vi "Read Stream Data File Multiple Channel.vi"() -> ()   [LabVIEW 2020]
panel:
  out "Array":dbl[][](array[numeric])
  in  "Channel":u64
  out "Waveform Graph":dbl[][](graph)
  in  "File Path":path
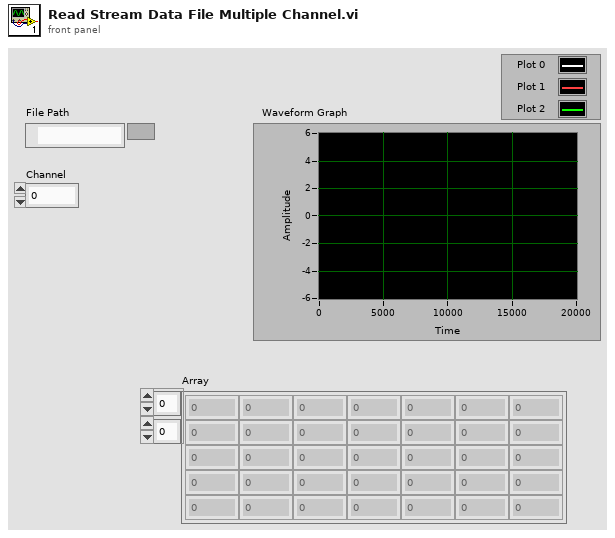
[diagram p1: front panel]
types:
  T1 = enum16{"open", "replace", "create", "open or create", "replace or create", "replace or create with confirmation"}
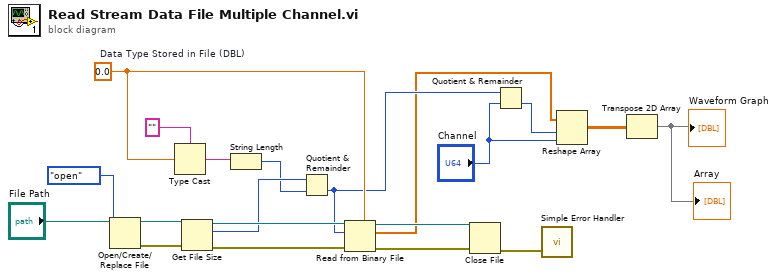
[diagram p0: block diagram]
diagram:
  w14 = 0.0  # Data Type Stored in File (DBL)
  n1 = Open/Create/Replace File(file path (use dialog)="File Path", operation (0:open)=T1."open") -> (refnum out=w18:refnum<file>, error out=w16:errorcluster)  [unwired: 4 in, 1 out]
  n2 = Type Cast(type="", x=w14) -> (*(type *) &x=w12:string)
  n3 = Get File Size(file=w18, error in=w16) -> (refnum out=w17:refnum<file>, size (in bytes)=w11:i64, 0:w15:errorcluster)
  n4 = String Length(string=w12) -> (length=w10:i32)
  n5 = Quotient & Remainder(x=w11, y=w10) -> (floor(x/y)=w6:i64)  [unwired: 1 out]
  n6 = Read from Binary File(5:w14, 8:w15, 10:w6, 11:w17) -> (0:w8:errorcluster, 2:w5:dbl[], 3:w9:refnum<file>)  [unwired: 2 in, 1 out]
  n7 = Close File(refnum=w9, error in=w8) -> (error out=w7:errorcluster)  [unwired: 1 out]
  n8 = Quotient & Remainder(x=w6, y="Channel") -> (floor(x/y)=w2:u64)  [unwired: 1 out]
  n9 = call <vilib>:"Simple Error Handler.vi"("error in (no error)"=w7) -> ()  [unwired: 4 in, 5 out]
  n10 = Reshape Array "Reshape Array"(w5, w2, "Channel") -> (w3:dbl[][])
  n11 = Transpose 2D Array(2D array=w3) -> (transposed array=→"Waveform Graph" →"Array":dbl[][])
